vi "GenNewTraj.vi"(10 "Parameters":T1, 11 "Points in":cluster{"x":dbl, "y":dbl, "th":dbl}[](array[cluster])) -> (0 "Time (s)":dbl, 1 "Valid":bool, 2 "Trajectory Data":T2(array[cluster]), 3 "Updated Waypoints":cluster{"x":dbl, "y":dbl, "th":dbl}[](array[cluster]), 4 "Distance (ft)":dbl)   [LabVIEW 2019]
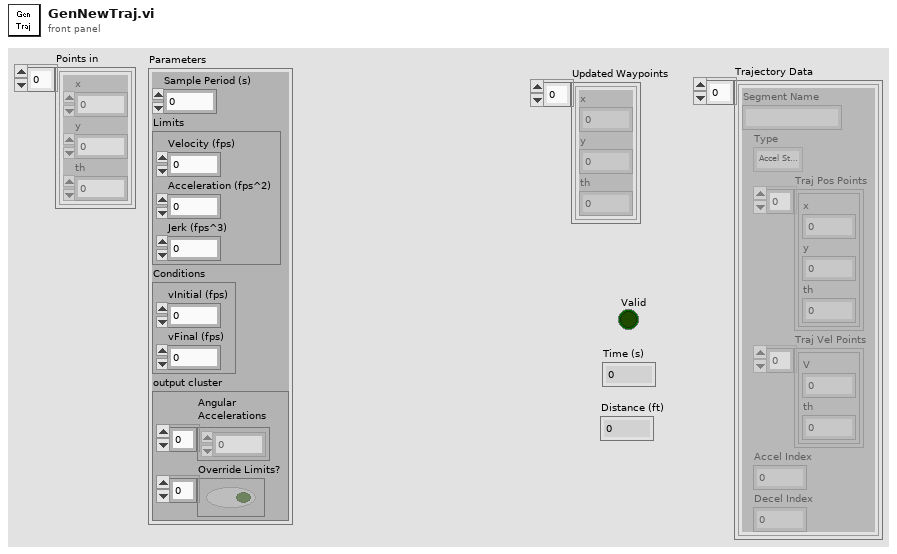
[diagram p1: front panel]
types:
  T1 = cluster{"Sample Period (s)":dbl, "Limits":cluster{"Velocity (fps)":dbl, "Acceleration (fps^2)":dbl, "Jerk (fps^3)":dbl}, "Conditions":cluster{"vInitial (fps)":dbl, "vFinal (fps)":dbl}, "output cluster":cluster{"Angular \nAccelerations":dbl[], "Override Limits?":bool[]}}
  T2 = cluster{"Segment Name":string, "Type":enum16{"Accel Straight", "Const Straight", "Blend", "Circle"}, "Traj Pos Points":cluster{"x":dbl, "y":dbl, "th":dbl}[], "Traj Vel Points":cluster{"V":dbl, "th":dbl}[], "Accel Index":i32, "Decel Index":i32}[]
  T3 = cluster{"Velocity (fps)":dbl, "Acceleration (fps^2)":dbl, "Jerk (fps^3)":dbl}
  T4 = cluster{"vInitial (fps)":dbl, "vFinal (fps)":dbl}
  T5 = cluster{"Angular \nAccelerations":dbl[], "Override Limits?":bool[]}
  T6 = cluster{"Trajectory Data":cluster{"Segment Name":string, "Type":enum16{"Accel Straight", "Const Straight", "Blend", "Circle"}, "Traj Pos Points":cluster{"x":dbl, "y":dbl, "th":dbl}[], "Traj Vel Points":cluster{"V":dbl, "th":dbl}[], "Accel Index":i32, "Decel Index":i32}[], "Time (s)":dbl, "Valid":bool, "Updated Waypoints":cluster{"x":dbl, "y":dbl, "th":dbl}[], "Distance (ft)":dbl}
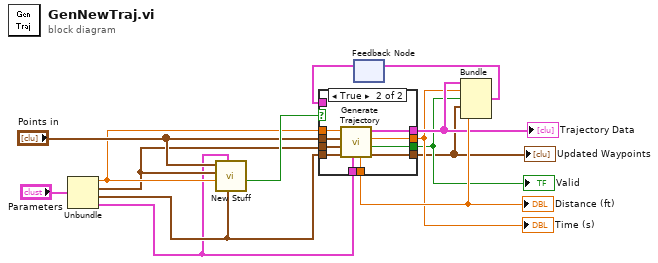
[diagram p0: block diagram]
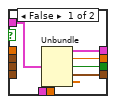
[diagram p2: hidden frame]
diagram:
  n1 = Unbundle("Parameters") -> ("Sample Period (s)"=w4:dbl, "Limits"=w3:T3, "Conditions"=w2:T4, "output cluster"=w1:T5)
  n2 = call "New Stuff.vi"("Conditions"=w2, "Angular Accelerations"=w1, "Sample Period (s)"=w4, "Limits"=w3, "Points in"="Points in") -> ("result"=w14:bool)  [unwired: 6 in]
  n3 = feedback #1() -> (w11:T6)  [unwired: 1 in]
  n4 = case shown="True" w14 {
    tunnel: [w17 w30] -> w7
    tunnel: [w18 w29] -> w8
    tunnel: [w15 w28] -> w13
    tunnel: w2 -> [_ w27]
    tunnel: w3 -> [_ w26]
    tunnel: w1 -> [_ w25]
    tunnel: "Points in" -> [_ w24]
    tunnel: [w16 w23] -> w6
    tunnel: [w19 w22] -> w9
    tunnel: w4 -> [_ w21]
    tunnel: w11 -> [w20 _]
    frame False {
      n5 = Unbundle(w20) -> ("Trajectory Data"=w19:T2, "Time (s)"=w18:dbl, "Valid"=w17:bool, "Updated Waypoints"=w16:cluster{"x":dbl, "y":dbl, "th":dbl}[], "Distance (ft)"=w15:dbl)
    }
    frame True {
      n6 = call "Generate Trajectory.vi"("Angular Accelerations"=w25, "Conditions"=w27, "Limits"=w26, "WayPoints"=w24, "Sample Period (s)"=w21) -> ("Updated Waypoints"=w23:cluster{"x":dbl, "y":dbl, "th":dbl}[], "Valid"=w30:bool, "Time (s)"=w29:dbl, "Trajectory Data"=w22:T2, "Distance (ft)"=w28:dbl)  [unwired: 2 in]
    }
  }
  "Distance (ft)" <- w13
  "Trajectory Data" <- w9
  "Time (s)" <- w8
  "Valid" <- w7
  "Updated Waypoints" <- w6
  n7 = Bundle("Trajectory Data"=w9, "Time (s)"=w8, "Valid"=w7, "Updated Waypoints"=w6, "Distance (ft)"=w13) -> (w10:T6)  [unwired: 1 in]
  n8 = feedback-in #1(w10) -> ()
